vi "RC_calibration_ver2.vi"(8 "error in (no error)":errorcluster, 10 "Motors IDs Found":u8[](array[numeric]), 11 "VISA resource name":refnum<visa-resource-name>) -> (0 "error out":errorcluster, 1 "Dynamixel Cycles":T1, 2 "output cluster":T2={"Main Dynamixel Set Data"={"Lower Winch Bound (deg)"=0.0, "Upper Winch Bound (deg)"=1000.0}, "Rudder Dynamixel Set Data"={"Lower Winch Bound (deg)"=30.0, "Upper Winch Bound (deg)"=90.0}, "Jib Dynamixel Set Data"={"Lower Winch Bound (deg)"=0.0, "Upper Winch Bound (deg)"=1000.0}}, 3 "VISA resource name out":refnum<visa-resource-name>)   [LabVIEW 2013]
doc: "Allows the user to set the maximum and minimum points for the sails and center the rudder. Necessary because the Dynamixels can't measure their position along the pulley system.\n\nTakes in the port the Dynamixels are plugged into and the indexes of the motors. Outputs the minimum and maximum points for all three motors and what cycle the motors are at when the code ends along with the port and any errors that occurred."
uses:
  Data/TypeDefs/MotorSetup.ctl
  Data/TypeDefs/DynamixelSetupInfo.ctl
  Data/TypeDefs/DynamixelCycleTracker.ctl
  <instrlib>/Dynamixel Motor/Dynamixel Motor.lvlib
panel:
  in  "Dynamixel Cycles Constant":T1
  in  "Rudder centered?":bool
  in  "Rudder offset":dbl=30.0
  in  "Set Rudder position":dbl=150.0
  out "Rudder position":dbl
  in  "Jib movement 2":dbl
  out "Jib offset from\nmin to max":dbl
  out "Jib position\nat max":dbl
  out "Jib rotations to max":i32
  in  "Jib at maximum?":bool
  out "Jib minimum":dbl
  in  "Jib at minimum?":bool
  in  "Jib movement 1":dbl
  in  "Main movement 2":dbl
  out "Main offset from\nmin to max":dbl
  out "Main position\nat max":dbl
  out "Main rotations to max":i32
  in  "Main at maximum?":bool
  out "Main minimum":dbl
  in  "Main at minimum?":bool
  in  "Main movement 1":dbl
  # "TODO: Check labels for main/jib are right"
  # "1. Arrow up/down on main movement 1\n     to have sails move toward all in\n2. When it is as far in as is safe (given \n    pulleys) hit \"Main at minimum\" button"
  # "3. Arrow up/down on main movement 2 \n    to have sails move toward all out\n4. When it is as far out as is safe (given \n    pulleys) hit \"Main at maximum\" button"
  # "5. Arrow up/down on jib movement 1\n     to have sails move toward all in\n6. When it is as far in as is safe (given\n    pulleys) hit \"Jib at minimum\" button"
  # "7. Arrow up/down on jib movement 2 \n    to have sails move toward all out\n8. When it is as far out as is safe (given\n    pulleys) hit \"Jib at maximum\" button"
  # "(as of 4/2/2014)\nSail 1 (main?, right if facing toward bow):\n+ speed goes in, makes position count down (including rotations)\n- speed goes out, makes position count up (including rotations)\nSail 2 (jib?, left if facing toward bow):\n+ speed goes out, makes position count down (including rotations)\n- speed goes in, makes position count up (including rotations)"
  # "9. Change rudder position until it is centered,\n     then hit \"rudder centered\"\n10. Set the offset from rudder center to min/max"
  # "Inputs/outputs you don't need to worry about"
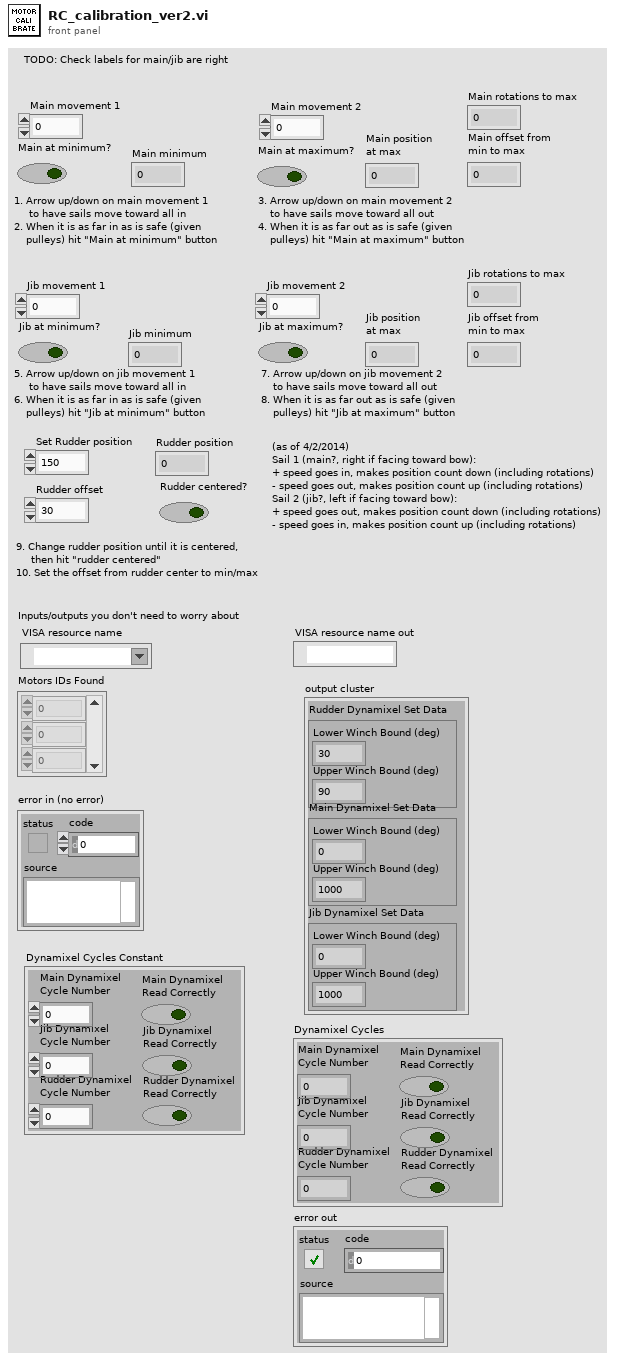
[diagram p1: front panel]
types:
  T1 = typedef "DynamixelCycleTracker.ctl" = cluster{"Main Dynamixel\nCycle Number":i32, "Jib Dynamixel\nCycle Number":i32, "Rudder Dynamixel\nCycle Number":i32, "Main Dynamixel\nRead Correctly":bool, "Jib Dynamixel\nRead Correctly":bool, "Rudder Dynamixel\nRead Correctly":bool}
  T2 = typedef "MotorSetup.ctl" = cluster{"Main Dynamixel Set Data":T3, "Rudder Dynamixel Set Data":T3, "Jib Dynamixel Set Data":T3}
  T3 = typedef "DynamixelSetupInfo.ctl" = cluster{"Lower Winch Bound (deg)":dbl, "Upper Winch Bound (deg)":dbl}
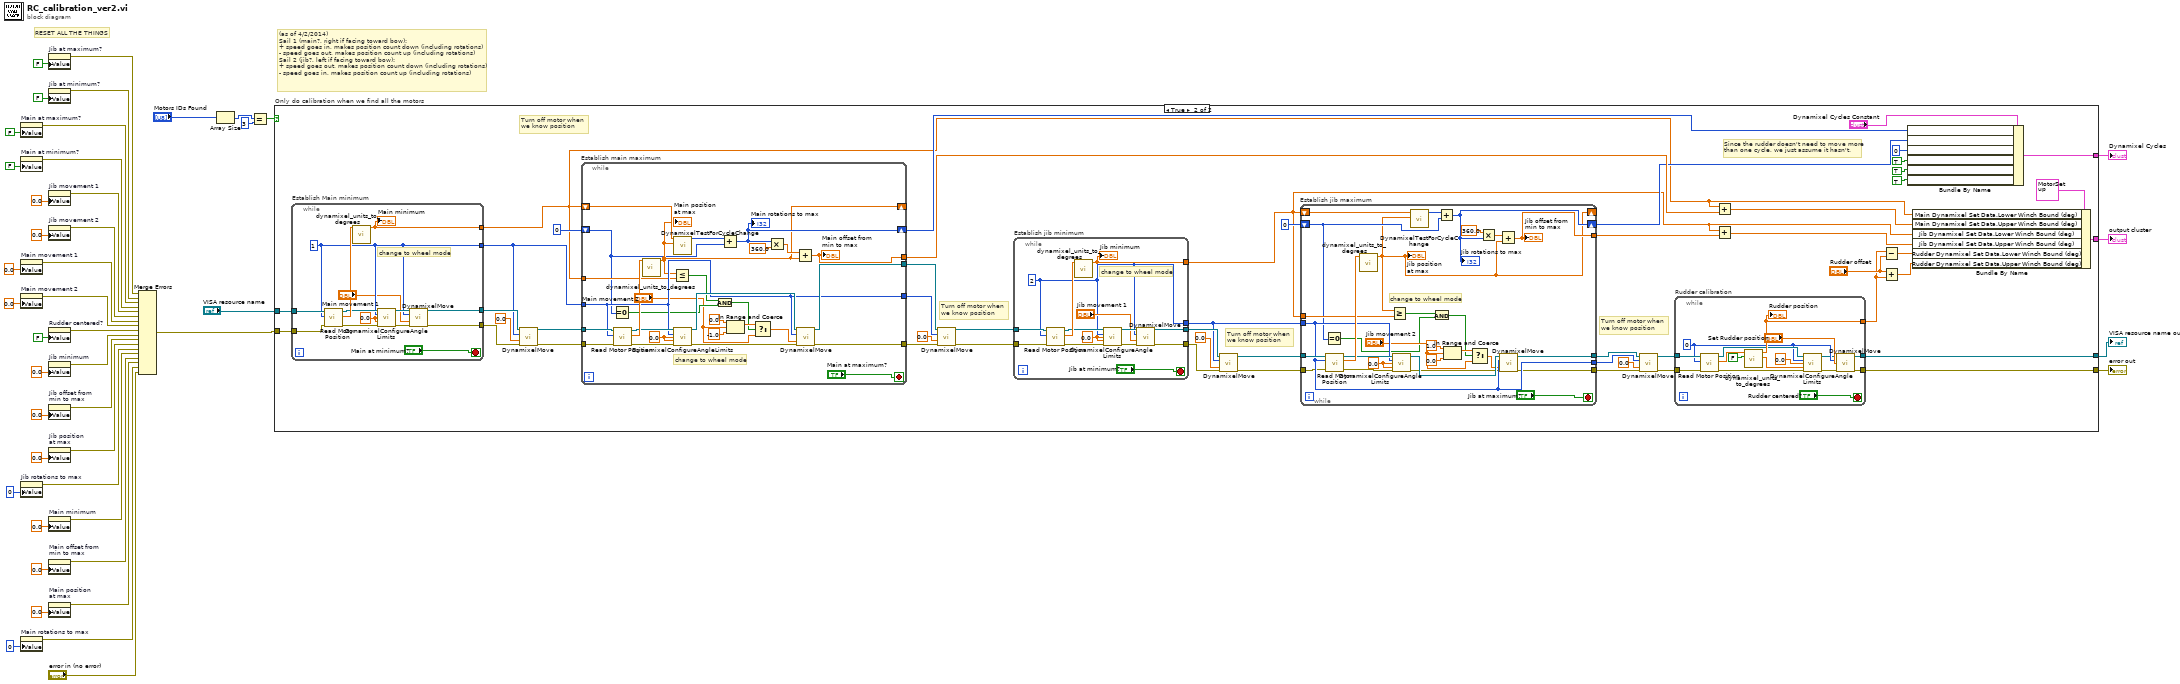
[diagram p0: block diagram]
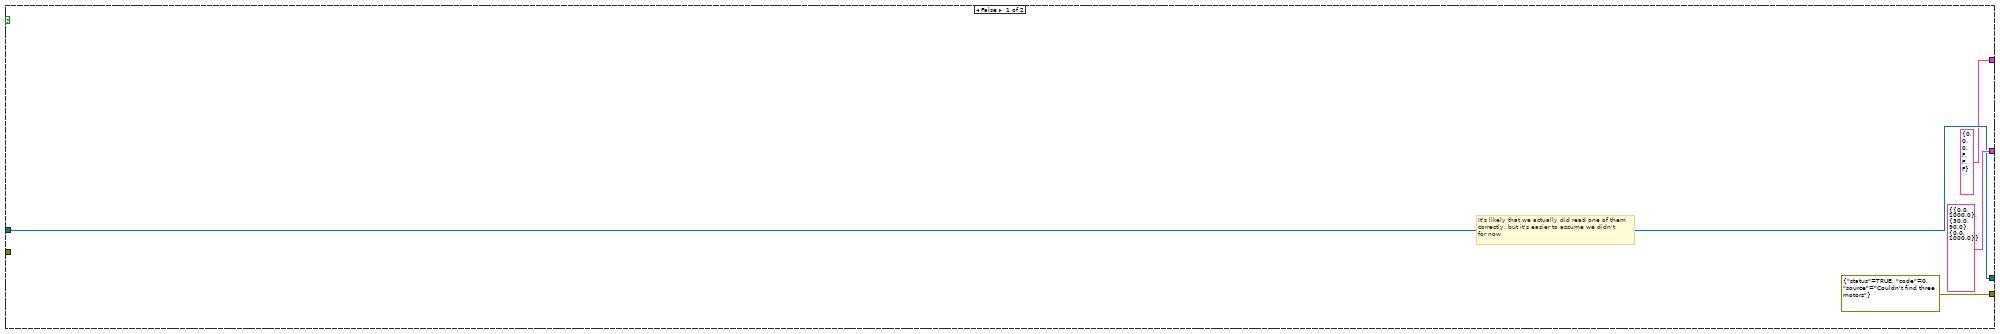
[diagram p2: hidden frame]
diagram:
  # "(as of 4/2/2014)\nSail 1 (main?, right if facing toward bow):\n+ speed goes in, makes position count down (including rotations)\n- speed goes out, makes position count up (including rotations)\nSail 2 (jib?, left if facing toward bow):\n+ speed goes out, makes position count down (including rotations)\n- speed goes in, makes position count up (including rotations)"
  # "RESET ALL THE THINGS"
  n1 = property on="Main at maximum?" class="Bool (strict)"("Value"=FALSE ("Main at maximum?")) -> (error out=w20:errorcluster)  [unwired: 2 in, 1 out]
  n2 = property on="Main at minimum?" class="Bool (strict)"("Value"=FALSE ("Main at minimum?")) -> (error out=w21:errorcluster)  [unwired: 2 in, 1 out]
  n3 = property on="Main movement 1" class="DigNum (strict)"("Value"=0.0 ("Main movement 1")) -> (error out=w24:errorcluster)  [unwired: 2 in, 1 out]
  n4 = property on="Main movement 2" class="DigNum (strict)"("Value"=0.0 ("Main movement 2")) -> (error out=w25:errorcluster)  [unwired: 2 in, 1 out]
  n5 = property on="Jib rotations to max" class="DigNum (strict)"("Value"=0 ("Jib rotations to max")) -> (error out=w6:errorcluster)  [unwired: 2 in, 1 out]
  n6 = property on="Main rotations to max" class="DigNum (strict)"("Value"=0 ("Main rotations to max")) -> (error out=w2:errorcluster)  [unwired: 2 in, 1 out]
  n7 = property on="Jib at maximum?" class="Bool (strict)"("Value"=FALSE ("Jib at maximum?")) -> (error out=w18:errorcluster)  [unwired: 2 in, 1 out]
  n8 = property on="Jib at minimum?" class="Bool (strict)"("Value"=FALSE ("Jib at minimum?")) -> (error out=w19:errorcluster)  [unwired: 2 in, 1 out]
  n9 = property on="Jib movement 1" class="DigNum (strict)"("Value"=0.0 ("Jib movement 1")) -> (error out=w22:errorcluster)  [unwired: 2 in, 1 out]
  n10 = property on="Jib movement 2" class="DigNum (strict)"("Value"=0.0 ("Jib movement 2")) -> (error out=w23:errorcluster)  [unwired: 2 in, 1 out]
  n11 = property on="Rudder centered?" class="Bool (strict)"("Value"=FALSE ("Rudder centered?")) -> (error out=w26:errorcluster)  [unwired: 2 in, 1 out]
  n12 = property on="Jib minimum" class="DigNum (strict)"("Value"=0.0 ("Jib minimum")) -> (error out=w9:errorcluster)  [unwired: 2 in, 1 out]
  n13 = property on="Jib offset from\nmin to max" class="DigNum (strict)"("Value"=0.0 ("Jib offset from\nmin to max")) -> (error out=w8:errorcluster)  [unwired: 2 in, 1 out]
  n14 = property on="Jib position\nat max" class="DigNum (strict)"("Value"=0.0 ("Jib position\nat max")) -> (error out=w7:errorcluster)  [unwired: 2 in, 1 out]
  n15 = property on="Main minimum" class="DigNum (strict)"("Value"=0.0 ("Main minimum")) -> (error out=w5:errorcluster)  [unwired: 2 in, 1 out]
  n16 = property on="Main offset from\nmin to max" class="DigNum (strict)"("Value"=0.0 ("Main offset from\nmin to max")) -> (error out=w4:errorcluster)  [unwired: 2 in, 1 out]
  n17 = property on="Main position\nat max" class="DigNum (strict)"("Value"=0.0 ("Main position\nat max")) -> (error out=w3:errorcluster)  [unwired: 2 in, 1 out]
  n18 = Merge Errors(w18, w19, w20, w21, w22, w23, w24, w25, w26, w9, w8, w7, w6, w5, w4, w3, w2, "error in (no error)") -> (w27:errorcluster)
  n19 = Array Size(array="Motors IDs Found") -> (size(s)=w43:i32)
  n20 = Equal?(x=w43, y=3) -> (x = y?=w33:bool)
  n21 = case "Only do calibration when we find all the motors" shown="True" w33 {
    tunnel: "VISA resource name" -> [w48 w99]
    tunnel: [T2 {"Main Dynamixel Set Data"={"Lower Winch Bound (deg)"=0.0, "Upper Winch Bound (deg)"=1000.0}, "Rudder Dynamixel Set Data"={"Lower Winch Bound (deg)"=30.0, "Upper Winch Bound (deg)"=90.0}, "Jib Dynamixel Set Data"={"Lower Winch Bound (deg)"=0.0, "Upper Winch Bound (deg)"=1000.0}} ("Dynamixel Bounds Control") w62] -> w44
    tunnel: [w48 w61] -> w40
    tunnel: w27 -> [_ w75]
    tunnel: [errorcluster {"status"=TRUE, "code"=0, "source"="Couldn't find three motors"} ("error out") w60] -> w39
    tunnel: [T1 {"Main Dynamixel\nCycle Number"=0, "Jib Dynamixel\nCycle Number"=0, "Rudder Dynamixel\nCycle Number"=0, "Main Dynamixel\nRead Correctly"=FALSE, "Jib Dynamixel\nRead Correctly"=FALSE, "Rudder Dynamixel\nRead Correctly"=FALSE} ("Dynamixel Cycles Constant") w58] -> w38
    frame False {
      # "It's likely that we actually did read one of them\ncorrectly, but it's easier to assume we didn't \nfor now"
    }
    frame True {
      # "Since the rudder doesn't need to move more\nthan one cycle, we just assume it hasn't."
      # "Turn off motor when \nwe know position"
      # "Turn off motor when \nwe know position"
      # "Turn off motor when \nwe know position"
      # "Turn off motor when \nwe know position"
      n22 = while "Establish Main minimum" {
        tunnel: w99 -> [w171]
        tunnel: [w169] -> w51
        tunnel: [w165] -> w98
        tunnel: [w164] -> w93
        tunnel: w75 -> [w163]
        tunnel: [w160] -> w74
        stop <- "Main at minimum?" stop-if-true
        w167 = 0.0 ("Clockwise Angle Limit (0 deg)")
        w164 = u8 1 ("Motor ID (0)")
        # "change to wheel mode"
        n23 = call <instrlib>:"Read Motor Position.vi"("error in (no error)"=w163, "Motor ID (0)"=w164, "VISA resource name"=w171) -> ("error out"=w162:errorcluster, "Position (deg)"=w170:dbl, "VISA resource name out"=w168:refnum<visa-resource-name>)  [unwired: 6 in]
        n24 = call "dynamixel_units_to_degrees.vi"("Dynamixel Input"=w170) -> ("Degrees"=w169:dbl)  [unwired: 9 in, 1 out]
        "Main minimum" <- w169
        n25 = call "DynamixelConfigureAngleLimits.vi"("VISA resource name"=w168, "Motor ID (0)"=w164, "Clockwise Angle Limit (0 deg)"=w167, "Counter-Clockwise Angle Limit (300 deg)"=w167, "error in (no error)"=w162) -> ("VISA resource name out"=w166:refnum<visa-resource-name>, "error out"=w161:errorcluster)  [unwired: 9 in]
        n26 = call "DynamixelMove.vi"("VISA resource name"=w166, "Motor ID (0)"=w164, "Goal Speed (RPM)"="Main movement 1", "error in (no error)"=w161) -> ("VISA resource name out"=w165:refnum<visa-resource-name>, "error out"=w160:errorcluster)  [unwired: 10 in]
      }
      n27 = call "DynamixelMove.vi"("VISA resource name"=w98, "Motor ID (0)"=w93, "Goal Speed (RPM)"=0.0, "error in (no error)"=w74) -> ("VISA resource name out"=w96:refnum<visa-resource-name>, "error out"=w73:errorcluster)  [unwired: 10 in]
      n28 = while "Establish main maximum" {
        tunnel: w96 -> [w201]
        tunnel: [w196] -> w94
        tunnel: w93 -> [w193]
        tunnel: [w193] -> w81
        tunnel: w73 -> [w192]
        tunnel: [w189] -> w72
        shift-right: [w175] -> _
        shift-left: w51 -> [w188]
        shift-right: [w184] -> w57
        shift-left: 0 ("Dynamixel Cycle Number") -> [w173]
        tunnel: [w185] -> w65
        tunnel: w51 -> [w176]
        stop <- "Main at maximum?" stop-if-true
        w198 = 0.0 ("Clockwise Angle Limit (0 deg)")
        # "change to wheel mode"
        n29 = Equal To 0?(x=w173) -> (x = 0?=w183:bool)
        n30 = call <instrlib>:"Read Motor Position.vi"("error in (no error)"=w192, "Motor ID (0)"=w193, "VISA resource name"=w201) -> ("error out"=w191:errorcluster, "Position (deg)"=w200:dbl, "VISA resource name out"=w199:refnum<visa-resource-name>)  [unwired: 6 in]
        n31 = call "dynamixel_units_to_degrees.vi"("Dynamixel Input"=w200) -> ("Degrees"=w175:dbl)  [unwired: 9 in, 1 out]
        "Main position\nat max" <- w175
        n32 = Less Or Equal?(x=w175, y=w176) -> (x <= y?=w174:bool)
        n33 = call "DynamixelTestForCycleChange.vi"("New position (deg)"=w175, "Old position (deg)"=w188) -> ("Dynamixel Cycle Number"=w186:i32)  [unwired: 9 in]
        n34 = call "DynamixelConfigureAngleLimits.vi"("VISA resource name"=w199, "Motor ID (0)"=w193, "Clockwise Angle Limit (0 deg)"=w198, "Counter-Clockwise Angle Limit (300 deg)"=w198, "error in (no error)"=w191) -> ("VISA resource name out"=w197:refnum<visa-resource-name>, "error out"=w190:errorcluster)  [unwired: 9 in]
        n35 = And(x=w174, y=w183) -> (x .and. y?=w179:bool)
        n36 = Add(x=w186, y=w173) -> (x+y=w184:i32)
        "Main rotations to max" <- w184
        n37 = In Range and Coerce(upper limit=0.0, x="Main movement 2", lower limit=-1.0) -> (coerced(x)=w182:dbl)  [unwired: 1 out]
        n38 = Select(t=w182, s=w179, f="Main movement 2") -> (s? t:f=w177:dbl)
        n39 = Multiply(x=w184, y=360.0) -> (x*y=w187:dbl)
        n40 = Add(x=w187, y=w175) -> (x+y=w185:dbl)
        "Main offset from\nmin to max" <- w185
        n41 = call "DynamixelMove.vi"("VISA resource name"=w197, "Motor ID (0)"=w193, "Goal Speed (RPM)"=w177, "error in (no error)"=w190) -> ("VISA resource name out"=w196:refnum<visa-resource-name>, "error out"=w189:errorcluster)  [unwired: 10 in]
      }
      n42 = call "DynamixelMove.vi"("VISA resource name"=w94, "Motor ID (0)"=w81, "Goal Speed (RPM)"=0.0, "error in (no error)"=w72) -> ("VISA resource name out"=w92:refnum<visa-resource-name>, "error out"=w71:errorcluster)  [unwired: 10 in]
      n43 = while "Establish jib minimum" {
        tunnel: w92 -> [w153]
        tunnel: [w151] -> w90
        tunnel: [w150] -> w50
        tunnel: [w149] -> w88
        tunnel: w71 -> [w148]
        tunnel: [w145] -> w70
        stop <- "Jib at minimum?" stop-if-true
        w155 = 0.0 ("Clockwise Angle Limit (0 deg)")
        w149 = u8 2 ("Motor ID (0)")
        # "change to wheel mode"
        n44 = call <instrlib>:"Read Motor Position.vi"("error in (no error)"=w148, "Motor ID (0)"=w149, "VISA resource name"=w153) -> ("error out"=w147:errorcluster, "Position (deg)"=w157:dbl, "VISA resource name out"=w156:refnum<visa-resource-name>)  [unwired: 6 in]
        n45 = call "dynamixel_units_to_degrees.vi"("Dynamixel Input"=w157) -> ("Degrees"=w150:dbl)  [unwired: 9 in, 1 out]
        "Jib minimum" <- w150
        n46 = call "DynamixelConfigureAngleLimits.vi"("VISA resource name"=w156, "Motor ID (0)"=w149, "Clockwise Angle Limit (0 deg)"=w155, "Counter-Clockwise Angle Limit (300 deg)"=w155, "error in (no error)"=w147) -> ("VISA resource name out"=w154:refnum<visa-resource-name>, "error out"=w146:errorcluster)  [unwired: 9 in]
        n47 = call "DynamixelMove.vi"("VISA resource name"=w154, "Motor ID (0)"=w149, "Goal Speed (RPM)"="Jib movement 1", "error in (no error)"=w146) -> ("VISA resource name out"=w151:refnum<visa-resource-name>, "error out"=w145:errorcluster)  [unwired: 10 in]
      }
      n48 = call "DynamixelMove.vi"("VISA resource name"=w90, "Motor ID (0)"=w88, "Goal Speed (RPM)"=0.0, "error in (no error)"=w70) -> ("VISA resource name out"=w89:refnum<visa-resource-name>, "error out"=w69:errorcluster)  [unwired: 10 in]
      n49 = while "Establish jib maximum" {
        tunnel: w89 -> [w139]
        tunnel: w88 -> [w137]
        tunnel: [w138] -> w86
        tunnel: [w137] -> w85
        tunnel: [w136] -> w76
        tunnel: w69 -> [w135]
        tunnel: [w132] -> w68
        shift-right: [w116] -> _
        shift-left: w50 -> [w131]
        shift-right: [w128] -> w56
        shift-left: 0 -> [w118]
        tunnel: w50 -> [w121]
        stop <- "Jib at maximum?" stop-if-true
        w142 = 0.0 ("Clockwise Angle Limit (0 deg)")
        # "change to wheel mode"
        n50 = Equal To 0?(x=w118) -> (x = 0?=w119:bool)
        n51 = call <instrlib>:"Read Motor Position.vi"("error in (no error)"=w135, "Motor ID (0)"=w137, "VISA resource name"=w139) -> ("error out"=w134:errorcluster, "Position (deg)"=w144:dbl, "VISA resource name out"=w143:refnum<visa-resource-name>)  [unwired: 6 in]
        n52 = call "dynamixel_units_to_degrees.vi"("Dynamixel Input"=w144) -> ("Degrees"=w116:dbl)  [unwired: 9 in, 1 out]
        "Jib position\nat max" <- w116
        n53 = Greater Or Equal?(x=w116, y=w121) -> (x >= y?=w120:bool)
        n54 = call "DynamixelConfigureAngleLimits.vi"("VISA resource name"=w143, "Motor ID (0)"=w137, "Clockwise Angle Limit (0 deg)"=w142, "Counter-Clockwise Angle Limit (300 deg)"=w142, "error in (no error)"=w134) -> ("VISA resource name out"=w141:refnum<visa-resource-name>, "error out"=w133:errorcluster)  [unwired: 9 in]
        n55 = call "DynamixelTestForCycleChange.vi"("New position (deg)"=w116, "Old position (deg)"=w131) -> ("Dynamixel Cycle Number"=w130:i32)  [unwired: 9 in]
        n56 = And(x=w120, y=w119) -> (x .and. y?=w124:bool)
        n57 = Add(x=w130, y=w118) -> (x+y=w128:i32)
        "Jib rotations to max" <- w128
        n58 = In Range and Coerce(upper limit=1.0, x="Jib movement 2", lower limit=0.0) -> (coerced(x)=w127:dbl)  [unwired: 1 out]
        n59 = Select(t=w127, s=w124, f="Jib movement 2") -> (s? t:f=w122:dbl)
        n60 = Multiply(x=360.0 ("y"), y=w128) -> (x*y=w117:dbl)
        n61 = Add(x=w117, y=w116) -> (x+y=w136:dbl)
        "Jib offset from\nmin to max" <- w136
        n62 = call "DynamixelMove.vi"("VISA resource name"=w141, "Motor ID (0)"=w137, "Goal Speed (RPM)"=w122, "error in (no error)"=w133) -> ("VISA resource name out"=w138:refnum<visa-resource-name>, "error out"=w132:errorcluster)  [unwired: 10 in]
      }
      n63 = call "DynamixelMove.vi"("VISA resource name"=w86, "Motor ID (0)"=w85, "Goal Speed (RPM)"=0.0, "error in (no error)"=w68) -> ("VISA resource name out"=w80:refnum<visa-resource-name>, "error out"=w67:errorcluster)  [unwired: 10 in]
      n64 = while "Rudder calibration" {
        tunnel: w80 -> [w115]
        tunnel: [w111] -> w63
        tunnel: [w110] -> w61
        tunnel: w67 -> [w109]
        tunnel: [w108] -> w60
        stop <- "Rudder centered?" stop-if-true
        w104 = u8 0 ("Motor ID (0)")
        n65 = call <instrlib>:"Read Motor Position.vi"("error in (no error)"=w109, "Motor ID (0)"=w104, "VISA resource name"=w115) -> ("error out"=w102:errorcluster, "Position (deg)"=w114:dbl, "VISA resource name out"=w106:refnum<visa-resource-name>)  [unwired: 6 in]
        n66 = call "dynamixel_units_to_degrees.vi"("MX Motor? (T)"=FALSE, "Dynamixel Input"=w114) -> ("Dynamixel units/cycle"=w105:dbl, "Degrees"=w111:dbl)  [unwired: 8 in]
        "Rudder position" <- w111
        n67 = call "DynamixelConfigureAngleLimits.vi"("VISA resource name"=w106, "Motor ID (0)"=w104, "Clockwise Angle Limit (0 deg)"=0.0, "Counter-Clockwise Angle Limit (300 deg)"=w105, "error in (no error)"=w102) -> ("VISA resource name out"=w100:refnum<visa-resource-name>, "error out"=w101:errorcluster)  [unwired: 9 in]
        n68 = call "DynamixelMove.vi"("VISA resource name"=w100, "Motor ID (0)"=w104, "Goal Position (150 deg)"="Set Rudder position", "error in (no error)"=w101) -> ("VISA resource name out"=w110:refnum<visa-resource-name>, "error out"=w108:errorcluster)  [unwired: 10 in]
      }
      n69 = Add(x=w51, y=w65) -> (x+y=w82:dbl)
      n70 = Add(x=w50, y=w76) -> (x+y=w83:dbl)
      n71 = Subtract(x=w63, y="Rudder offset") -> (x-y=w79:dbl)
      n72 = Add(x="Rudder offset", y=w63) -> (x+y=w77:dbl)
      n73 = Bundle By Name(cluster="Dynamixel Cycles Constant", "Main Dynamixel\nCycle Number"=w57, "Jib Dynamixel\nCycle Number"=w56, "Rudder Dynamixel\nCycle Number"=0 ("Rudder Dynamixel\nCycle Number"), "Main Dynamixel\nRead Correctly"=TRUE ("Main Dynamixel\nRead Correctly"), "Jib Dynamixel\nRead Correctly"=TRUE ("Jib Dynamixel\nRead Correctly"), "Rudder Dynamixel\nRead Correctly"=TRUE ("Rudder Dynamixel\nRead Correctly")) -> (w58:T1)
      n74 = Bundle By Name(cluster=T2 {"Main Dynamixel Set Data"={"Lower Winch Bound (deg)"=122.55131964809384, "Upper Winch Bound (deg)"=922.5513196480938}, "Rudder Dynamixel Set Data"={"Lower Winch Bound (deg)"=15.0, "Upper Winch Bound (deg)"=60.0}, "Jib Dynamixel Set Data"={"Lower Winch Bound (deg)"=241.0557184750733, "Upper Winch Bound (deg)"=1041.0557184750733}} ("Dynamixel Bounds Control"), "Main Dynamixel Set Data.Lower Winch Bound (deg)"=w51, "Main Dynamixel Set Data.Upper Winch Bound (deg)"=w82, "Jib Dynamixel Set Data.Lower Winch Bound (deg)"=w50, "Jib Dynamixel Set Data.Upper Winch Bound (deg)"=w83, "Rudder Dynamixel Set Data.Lower Winch Bound (deg)"=w79, "Rudder Dynamixel Set Data.Upper Winch Bound (deg)"=w77) -> (w62:T2)
    }
  }
  "output cluster" <- w44
  "VISA resource name out" <- w40
  "error out" <- w39
  "Dynamixel Cycles" <- w38
